vi "Update Listbox.vi"(8 "error in (no error)":errorcluster, 9 "New Items":string[](array[string]), 10 "All Items":string[](array[string]), 11 "ListBox in":refnum<vi>) -> (0 "error out":errorcluster)   [LabVIEW 2020, in "Debugger.lvclass"]
uses:
  Debugger.lvclass
  Debugger.lvclass/Debugger.ctl
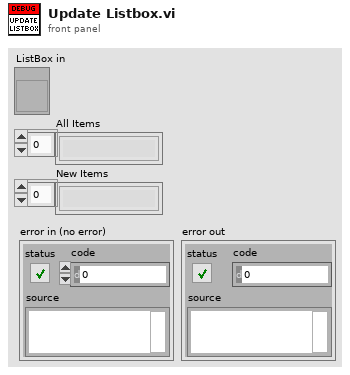
[diagram p1: front panel]
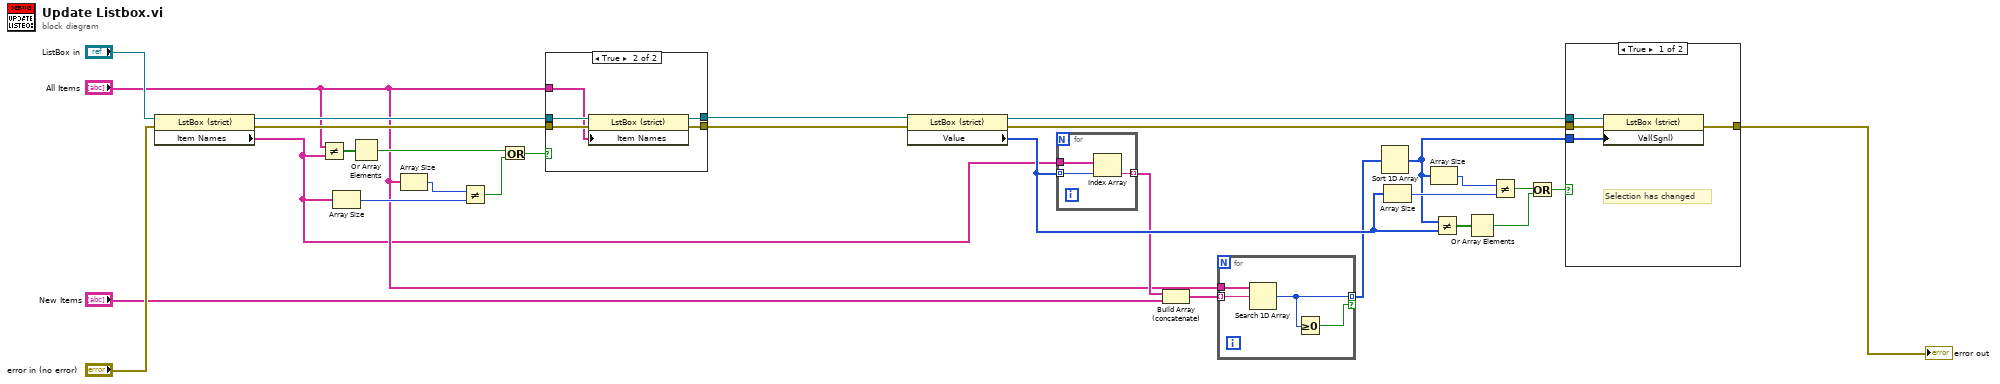
[diagram p0: block diagram]
diagram:
  n1 = property on="Property Node" class="LstBox (strict)"(reference="ListBox in", error in="error in (no error)") -> (reference out=w29:refnum<vi>, error out=w27:errorcluster, "Item Names"=w1:string[])
  n2 = Not Equal?(x="All Items", y=w1) -> (x != y?=w25:bool[])
  n3 = Array Size(array=w1) -> (size(s)=w24:i32)
  n4 = Or Array Elements(Boolean array=w25) -> (logical OR=w21:bool)
  n5 = Array Size(array="All Items") -> (size(s)=w23:i32)
  n6 = Not Equal?(x=w23, y=w24) -> (x != y?=w22:bool)
  n7 = Or(x=w21, y=w22) -> (x .or. y?=w20:bool)
  n8 = case shown="True" w20 {
    tunnel: w27 -> [w31 w36]
    tunnel: w29 -> [w30 w35]
    tunnel: [w31 w34] -> w4
    tunnel: "All Items" -> [_ w33]
    tunnel: [w30 w32] -> w5
    frame False {
    }
    frame True {
      n9 = property on="Property Node" class="LstBox (strict)"(reference=w35, error in=w36, "Item Names"=w33) -> (reference out=w32:refnum<vi>, error out=w34:errorcluster)
    }
  }
  n10 = property on="Property Node" class="LstBox (strict)"(reference=w5, error in=w4) -> (reference out=w8:refnum<vi>, error out=w9:errorcluster, "Value"=w14:i32[])
  n11 = for {
    tunnel: w1 -> [w39]
    tunnel: w14 -> [w38] mode=indexing
    tunnel: [w37] -> w11 mode=indexing
    n12 = Index Array(array=w39, index=w38) -> (element=w37:string)
  }
  n13 = Build Array (concatenate)(w11, "New Items") -> (w10:string[])
  n14 = for {
    tunnel: w10 -> [w42] mode=indexing
    tunnel: "All Items" -> [w43]
    tunnel: [w41] -> w7 mode=indexing if=w40
    n15 = Search 1D Array(1D array=w43, element=w42) -> (index of element=w41:i32)  [unwired: 1 in]
    n16 = Greater Or Equal To 0?(x=w41) -> (x >= 0?=w40:bool)
  }
  n17 = Sort 1D Array(array=w7) -> (sorted array=w13:i32[])
  n18 = Array Size(array=w14) -> (size(s)=w17:i32)
  n19 = Array Size(array=w13) -> (size(s)=w16:i32)
  n20 = Not Equal?(x=w13, y=w14) -> (x != y?=w12:bool[])
  n21 = Or Array Elements(Boolean array=w12) -> (logical OR=w18:bool)
  n22 = Not Equal?(x=w16, y=w17) -> (x != y?=w15:bool)
  n23 = Or(x=w15, y=w18) -> (x .or. y?=w19:bool)
  n24 = case shown="True" w19 {
    tunnel: w8 -> [w47 _]
    tunnel: w9 -> [w46 w48]
    tunnel: [w45 w48] -> w3
    tunnel: w13 -> [w44 _]
    frame True {
      # "Selection has changed"
      n25 = property on="Property Node" class="LstBox (strict)"(reference=w47, error in=w46, "Val(Sgnl)"=w44) -> (error out=w45:errorcluster)  [unwired: 1 out]
    }
    frame False {
    }
  }
  "error out" <- w3
